vi "PAM uPa per Volts.vi"() -> ()   [LabVIEW 2020, in "PAM Library.lvlib"]
uses:
  PAM Library.lvlib
panel:
  out "uPa per Volts":dbl
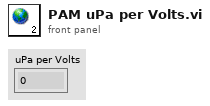
[diagram p1: front panel]
diagram:
